vi "CursorDraw_3_cursorView.vi"(8 "error in (no error)":errorcluster, 9 "Pos":cluster{"x":i16, "y":i16}, 10 "pict in":picture, 11 "Gviewer in":refnum<class "Gviewer.lvclass">) -> (0 "error out":errorcluster, 2 "pict out":picture, 3 "Gviewer out":refnum<class "Gviewer.lvclass">)   [LabVIEW 2020, in "Sgraph_lib_V1.lvlib" / "Gviewer.lvclass"]
doc: "Draw cursors and enable identification of a specific trace so it can be selected (s)"
uses:
  Gviewer.lvclass
  Gviewer.lvclass/Gviewer.ctl
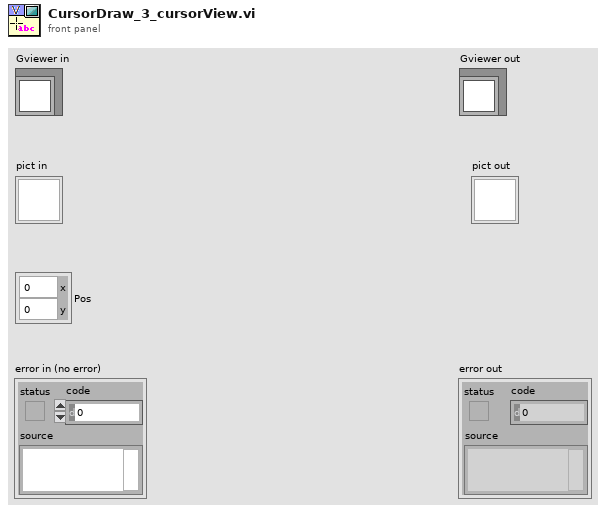
[diagram p1: front panel]
types:
  T1 = typedef "LVPoint32TypeDef.ctl" = cluster{"Horizontal":i32, "Vertical":i32}
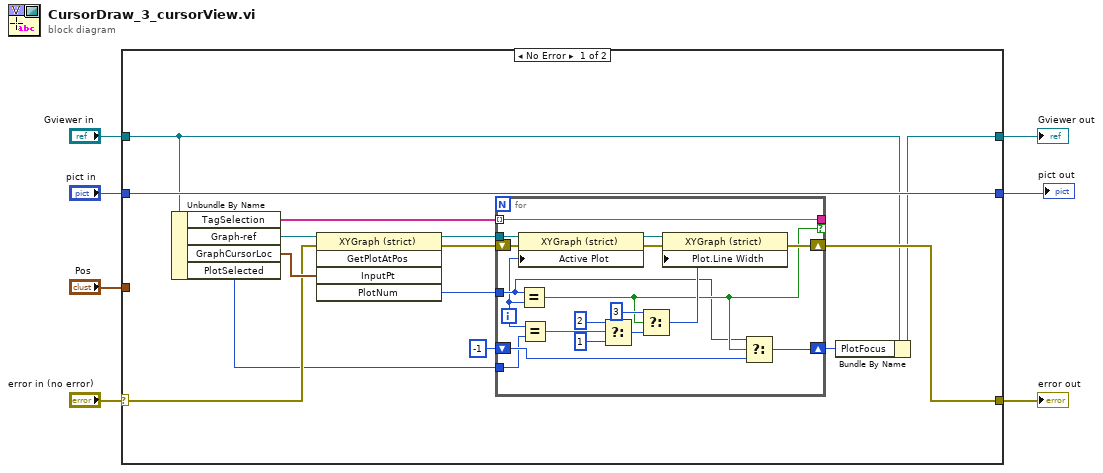
[diagram p0: block diagram]
diagram:
  n1 = case shown="No Error" "error in (no error)" {
    selector: "error in (no error)" -> [w18 w42]
    tunnel: [w13 w42] -> w6
    tunnel: [w10 w41] -> w4
    tunnel: "Gviewer in" -> [w9 w41]
    tunnel: "pict in" -> [w21 w40]
    tunnel: [w21 w40] -> w2
    tunnel: "Pos" -> [_ _]
    frame No Error {
      n2 = Unbundle By Name(w9) -> ("TagSelection"=w17:string[], "Graph-ref"=w20:refnum<vi>, "GraphCursorLoc"=w19:T1, "PlotSelected"=w8:i32)
      n3 = invoke class="XYGraph (strict)" method="GetPlotAtPos"(reference=w20, error in=w18, "InputPt"=w19) -> (reference out=w15:refnum<vi>, error out=w14:errorcluster, "PlotNum"=w16:i32)  [unwired: 2 in, 2 out]
      n4 = for {
        tunnel: w17 -> [w39] mode=indexing
        tunnel: w16 -> [w28]
        tunnel: [w39] -> _ if=w31
        tunnel: w15 -> [w38]
        shift-right: [w32] -> w13
        shift-left: w14 -> [w34]
        shift-right: [w29] -> w11
        shift-left: -1 -> [w30]
        tunnel: w8 -> [w25]
        i -> [w26]
        n5 = property class="XYGraph (strict)"(reference=w38, error in=w34, "Active Plot"=w26) -> (reference out=w37:refnum<vi>, error out=w33:errorcluster)
        n6 = Equal?(x=w28, y=w26) -> (x = y?=w31:bool)
        n7 = Equal?(x=w26, y=w25) -> (x = y?=w24:bool)
        n8 = Select(t=u8 2 ("Plot.Line Width"), s=w24, f=u8 1 ("Plot.Line Width")) -> (s? t:f=w27:u8)
        n9 = Select(t=u8 3 ("Plot.Line Width"), s=w31, f=w27) -> (s? t:f=w35:u8)
        n10 = property class="XYGraph (strict)"(reference=w37, error in=w33, "Plot.Line Width"=w35) -> (error out=w32:errorcluster)  [unwired: 1 out]
        n11 = Select(t=w28, s=w31, f=w30) -> (s? t:f=w29:i32)
      }
      n12 = Bundle By Name(cluster=w9, "PlotFocus"=w11) -> (w10:refnum<class "Gviewer.lvclass">)
    }
    frame Error {
    }
  }
  "error out" <- w6
  "Gviewer out" <- w4
  "pict out" <- w2
